vi "Read text with offset.vi"(6 "Count":i32, 7 "File Size":i64, 8 "Error In":errorcluster, 9 "Start of read offset (chars.: 0)":i64, 11 "Refnum In":refnum<file>) -> (0 "Error out":errorcluster, 1 "Mark after Read":i64, 2 "text":string, 3 "refnum out":refnum<file>, 4 "EOF?":bool)   [LabVIEW 2018]
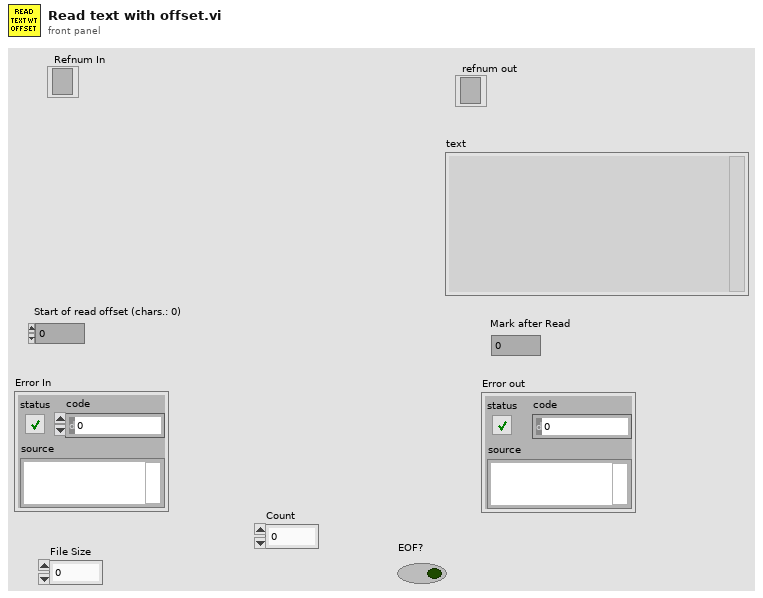
[diagram p1: front panel]
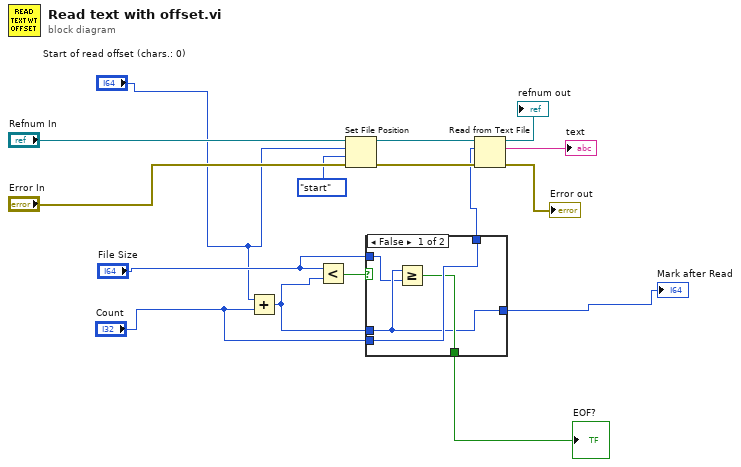
[diagram p0: block diagram]
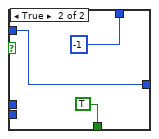
[diagram p2: hidden frame]
diagram:
  n1 = Add(x="Start of read offset (chars.: 0)", y="Count") -> (x+y=w6:i64)
  n2 = Less?(x="File Size", y=w6) -> (x < y?=w9:bool)
  n3 = Set File Position(offset (in bytes) (0)="Start of read offset (chars.: 0)", refnum="Refnum In", from (0:start)=enum16{"start", "end", "current"}."start", error in="Error In") -> (refnum out=w16:refnum<file>, error out=w15:errorcluster)
  n4 = case shown="False" w9 {
    tunnel: [w20 -1 ("t")] -> w3
    tunnel: [w18 w22] -> w8
    tunnel: "File Size" -> [w17 w22]
    tunnel: w6 -> [w18 _]
    tunnel: "Count" -> [w20 _]
    tunnel: [w19 TRUE] -> w1
    frame False {
      n5 = Greater Or Equal?(x=w18, y=w17) -> (x >= y?=w19:bool)
    }
    frame True {
    }
  }
  "Mark after Read" <- w8
  "EOF?" <- w1
  n6 = Read from Text File(file (use dialog)=w16, count=w3, error in=w15) -> (refnum out=→"refnum out":refnum<file>, text=→"text":string, error out=→"Error out":errorcluster)  [unwired: 1 in, 1 out]
